vi "Handle Help.vi"(8 "error in (no error)":errorcluster, 10 "Command":variant, 11 "Instrument in":refnum<class "Instrument.lvclass">) -> (0 "error out":errorcluster, 2 "Help":variant, 3 "Instrument out":refnum<class "Instrument.lvclass">)   [LabVIEW 2019, in "Instrument.lvlib" / "Instrument.lvclass"]
uses:
  Instrument.lvclass
  Typedefs/Instrument.HELP--Cluster.ctl
  5ed4e349-e1aa-442e-8035-ab7e90039f4b.vi
  ae75fb4e-d74c-4d65-9027-d3e49d8ff0d1.vi
  5ed4e349-e1aa-442e-8035-ab7e90039f4b.vi/71fe7c5d-2a80-4db2-ac7d-2e1464f569b6.vi
  5ed4e349-e1aa-442e-8035-ab7e90039f4b.vi/8746a56c-21ff-4136-bafd-1256caf14490.vi
  ae75fb4e-d74c-4d65-9027-d3e49d8ff0d1.vi/f6bf00ad-5039-4e74-a150-6496b52e5894.vi
  ae75fb4e-d74c-4d65-9027-d3e49d8ff0d1.vi/fae0fccd-bcc9-4717-a231-4d3b201867ff.vi
  <vilib>/Utility/Data Type/Get Type Information.vi
  <vilib>/JDP Science/JSONtext/JSON text to Variant.vi
  <vilib>/JDP Science/JSONtext/LVClass Serializer/JSONtext LVClass Serializer.lvclass
  subsystems/Help/Help.lvclass
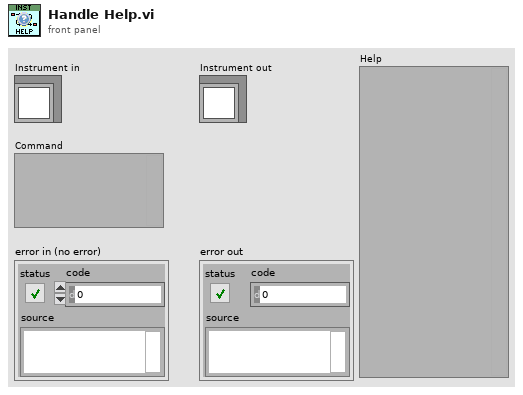
[diagram p1: front panel]
types:
  T1 = typedef "Instrument.lvlib/Instrument.lvclass/Instrument.HELP--Cluster.ctl" = cluster{"command":string}
  T2 = typedef "Instrument.lvlib/Help.lvclass/Help--cluster.ctl" = cluster{"command":string, "command description":string, "request cluster":variant, "response cluster":variant}
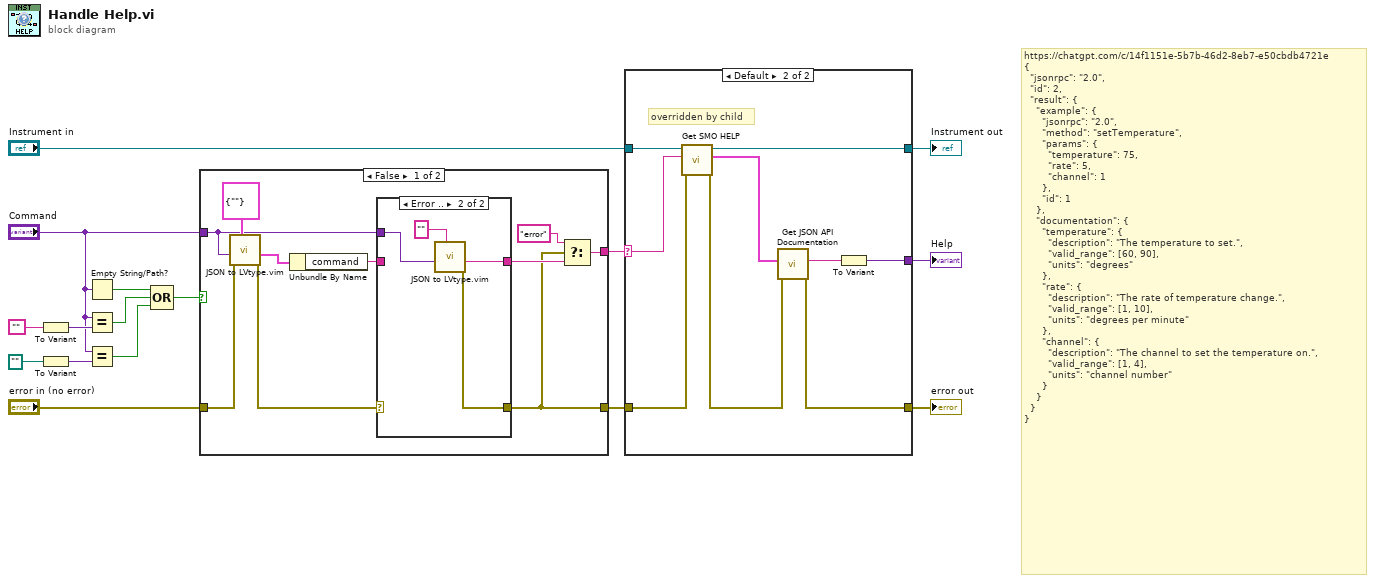
[diagram p0: block diagram]
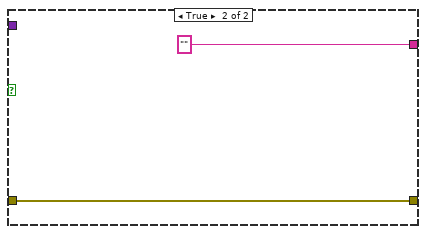
[diagram p3: hidden frame]
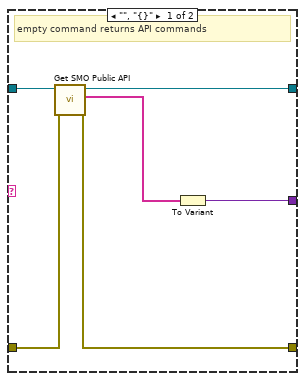
[diagram p4: hidden frame]
diagram:
  # "https://chatgpt.com/c/14f1151e-5b7b-46d2-8eb7-e50cbdb4721e\n{\n  \"jsonrpc\": \"2.0\",\n  \"id\": 2,\n  \"result\": {\n    \"example\": {\n      \"jsonrpc\": \"2.0\",\n      \"method\": \"setTemperature\",\n      \"params\": {\n        \"temperature\": 75,\n        \"rate\": 5,\n        \"channel\": 1\n      },\n      \"id\": 1\n    },\n    \"documentation\": {\n      \"temperature\": {\n        \"description\": \"The temperature to set.\",\n        \"valid_range\": [60, 90],\n        \"units\": \"degrees\"\n      },\n      \"rate\": {\n        \"description\": \"The rate of temperature change.\",\n        \"valid_range\": [1, 10],\n        \"units\": \"degrees per minute\"\n      },\n      \"channel\": {\n        \"description\": \"The channel to set the temperature on.\",\n        \"valid_range\": [1, 4],\n        \"units\": \"channel number\"\n      }\n    }\n  }\n}"
  n1 = To Variant(anything="") -> (Variant=w5:variant)
  n2 = To Variant(anything=path "") -> (Variant=w7:variant)
  n3 = Empty String/Path?(string/path="Command") -> (empty?=w6:bool)
  n4 = Equal?(x="Command", y=w5) -> (x = y?=w1:bool)
  n5 = Equal?(x="Command", y=w7) -> (x = y?=w2:bool)
  n6 = Compound Arithmetic op=OR(w6, w1, w2) -> (w3:bool)
  n7 = case shown="False" w3 {
    tunnel: "error in (no error)" -> [w26 w34]
    tunnel: [w25 ""] -> w13
    tunnel: [w17 w34] -> w14
    tunnel: "Command" -> [w18 _]
    frame False {
      n8 = call "JSON to LVtype.vim"("type"=T1 {"command"=""} ("Cluster"), "error in (no error)"=w26, "JSON Data in"=w18) -> ("error out"=w21:errorcluster, "Data out"=w22:T1)  [unwired: 7 in]
      n9 = Unbundle By Name(w22) -> ("command"=w19:string)
      n10 = case shown="Error .." w21 {
        selector: w21 -> [w28 _]
        tunnel: [w28 w30] -> w17
        tunnel: [w27 w29] -> w20
        tunnel: w19 -> [w27 _]
        tunnel: w18 -> [_ w31]
        frame No Error {
        }
        frame Error {
          n11 = call "JSON to LVtype.vim"("type"="", "JSON Data in"=w31) -> ("error out"=w30:errorcluster, "Data out"=w29:string)  [unwired: 8 in]
        }
      }
      n12 = Select(t="error", s=w17, f=w20) -> (s? t:f=w25:string)
    }
    frame True {
    }
  }
  n13 = case shown="Default" w13 {
    selector: w13 -> [_ w43]
    tunnel: w14 -> [w36 w45]
    tunnel: [w40 w48] -> w12
    tunnel: [w37 w41] -> w11
    tunnel: "Instrument in" -> [w39 w47]
    tunnel: [w35 w46] -> w10
    frame "", "{}" {
      # "empty command returns API commands"
      n14 = call-dynamic "Get SMO Public API.vi"("error in (no error)"=w36, "Instrument in"=w39) -> ("error out"=w37:errorcluster, "commands"=w38:string[], "Instrument out"=w35:refnum<class "Instrument.lvclass">)  [unwired: 7 in]
      n15 = To Variant(anything=w38) -> (Variant=w40:variant)
    }
    frame Default {
      # "overridden by child"
      n16 = call-dynamic "Get SMO HELP.vi"("error in (no error)"=w45, "Command"=w43, "Instrument in"=w47) -> ("error out"=w44:errorcluster, "help cluster"=w42:T2, "Instrument out"=w46:refnum<class "Instrument.lvclass">)  [unwired: 6 in]
      n17 = call "Get JSON API Documentation.vi"("error in (no error)"=w44, "Help cluster"=w42) -> ("error out"=w41:errorcluster, "<JSON> API doc"=w49:string)  [unwired: 7 in, 1 out]
      n18 = To Variant(anything=w49) -> (Variant=w48:variant)
    }
  }
  "Help" <- w12
  "Instrument out" <- w10
  "error out" <- w11
